vi "Vortex_AE.vi"(7 "Action":enum16{"READ", "WRITE"}(ring), 10 "Vortex In":dbl[][](array[numeric])) -> (2 "Vortex Out":dbl[][](array[numeric]))   [LabVIEW 2018]
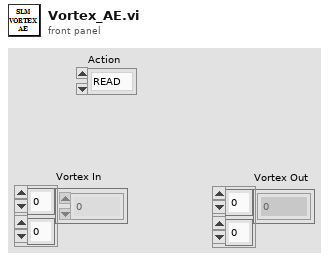
[diagram p1: front panel]
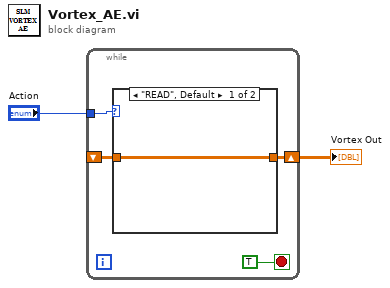
[diagram p0: block diagram]
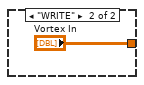
[diagram p2: hidden frame]
diagram:
  n1 = while {
    tunnel: "Action" -> [w5]
    shift-right: [w4] -> w1
    shift-left: _ -> [w3]
    stop <- TRUE stop-if-true
    n2 = case shown="\"READ\", Default" w5 {
      tunnel: [w7 "Vortex In"] -> w4
      tunnel: w3 -> [w7 _]
      frame "READ", Default {
      }
      frame "WRITE" {
      }
    }
  }
  "Vortex Out" <- w1
